vi "Mezclador.vi"() -> ()   [LabVIEW 2020]
panel:
  out "Mezclador":bool
  # "On=Enciende Mezclador\nOFF=Apaga mezclador"
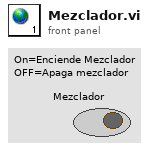
[diagram p1: front panel]
diagram:
